vi "AverageScanivalveValues.vi"(11 "Px Array":sgl[][](array[numeric])) -> (3 "Array":dbl[](array[numeric]))   [LabVIEW 2019]
uses:
  <vilib>/Analysis/baseanly.llb/Mean (DBL).vi
  <vilib>/Analysis/NI_AALBase.lvlib
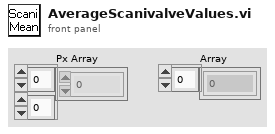
[diagram p1: front panel]
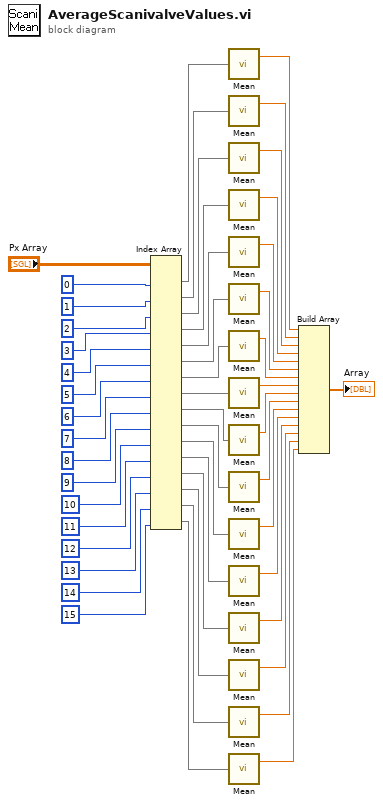
[diagram p0: block diagram]
diagram:
  n1 = Index Array(array="Px Array", index (col) #1=0 ("disabled index (col)"), index (col) #2=1 ("index (col)"), index (col) #3=2 ("index (col)"), index (col) #4=3 ("index (col)"), index (col) #5=4 ("index (col)"), index (col) #6=5 ("index (col)"), index (col) #7=6 ("index (col)"), index (col) #8=7 ("index (col)"), index (col) #9=8 ("index (col)"), index (col) #10=9 ("index (col)"), index (col) #11=10 ("index (col)"), index (col) #12=11 ("index (col)"), index (col) #13=12 ("index (col)"), index (col) #14=13 ("index (col)"), index (col) #15=14 ("index (col)"), index (col) #16=15 ("index (col)")) -> (element #1=w19:sgl[], element #2=w20:sgl[], element #3=w21:sgl[], element #4=w22:sgl[], element #5=w23:sgl[], element #6=w24:sgl[], element #7=w25:sgl[], element #8=w26:sgl[], element #9=w27:sgl[], element #10=w28:sgl[], element #11=w29:sgl[], element #12=w30:sgl[], element #13=w31:sgl[], element #14=w32:sgl[], element #15=w33:sgl[], element #16=w34:sgl[])  [unwired: 16 in]
  n2 = call-poly <vilib>:"Mean.vi"("X"=w19) -> ("mean"=w35:dbl)  [unwired: 1 out]
  n3 = call-poly <vilib>:"Mean.vi"("X"=w20) -> ("mean"=w36:dbl)  [unwired: 1 out]
  n4 = call-poly <vilib>:"Mean.vi"("X"=w21) -> ("mean"=w37:dbl)  [unwired: 1 out]
  n5 = call-poly <vilib>:"Mean.vi"("X"=w22) -> ("mean"=w38:dbl)  [unwired: 1 out]
  n6 = call-poly <vilib>:"Mean.vi"("X"=w23) -> ("mean"=w39:dbl)  [unwired: 1 out]
  n7 = call-poly <vilib>:"Mean.vi"("X"=w24) -> ("mean"=w40:dbl)  [unwired: 1 out]
  n8 = call-poly <vilib>:"Mean.vi"("X"=w25) -> ("mean"=w41:dbl)  [unwired: 1 out]
  n9 = call-poly <vilib>:"Mean.vi"("X"=w26) -> ("mean"=w42:dbl)  [unwired: 1 out]
  n10 = call-poly <vilib>:"Mean.vi"("X"=w27) -> ("mean"=w43:dbl)  [unwired: 1 out]
  n11 = call-poly <vilib>:"Mean.vi"("X"=w28) -> ("mean"=w44:dbl)  [unwired: 1 out]
  n12 = call-poly <vilib>:"Mean.vi"("X"=w29) -> ("mean"=w45:dbl)  [unwired: 1 out]
  n13 = call-poly <vilib>:"Mean.vi"("X"=w30) -> ("mean"=w46:dbl)  [unwired: 1 out]
  n14 = call-poly <vilib>:"Mean.vi"("X"=w31) -> ("mean"=w47:dbl)  [unwired: 1 out]
  n15 = call-poly <vilib>:"Mean.vi"("X"=w32) -> ("mean"=w48:dbl)  [unwired: 1 out]
  n16 = call-poly <vilib>:"Mean.vi"("X"=w33) -> ("mean"=w49:dbl)  [unwired: 1 out]
  n17 = call-poly <vilib>:"Mean.vi"("X"=w34) -> ("mean"=w50:dbl)  [unwired: 1 out]
  n18 = Build Array(w35, w36, w37, w38, w39, w40, w41, w42, w43, w44, w45, w46, w47, w48, w49, w50) -> (→"Array":dbl[])
